vi "Populate Graph Channel Names.vi"(8 "error in (no error)":errorcluster, 10 "Array":string[](array[string]), 11 "WaveformGraph in":refnum<vi>) -> (0 "error out":errorcluster, 3 "WaveformGraph out":refnum<vi>)   [LabVIEW 2015, in "Utility.lvlib"]
uses:
  Utility.lvlib
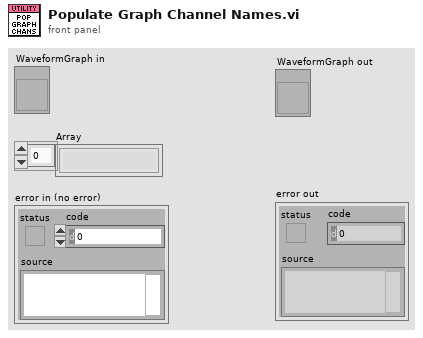
[diagram p1: front panel]
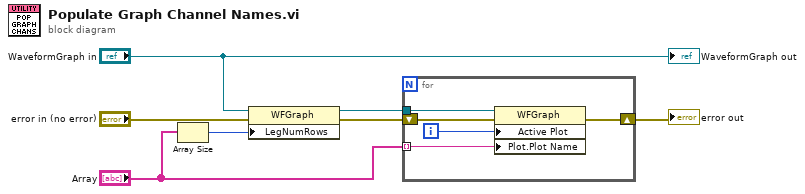
[diagram p0: block diagram]
diagram:
  n1 = Array Size(array="Array") -> (size(s)=w7:i32)
  n2 = property class="WFGraph"(reference="WaveformGraph in", error in="error in (no error)", "LegNumRows"=w7) -> (reference out=w5:refnum<vi>, error out=w3:errorcluster)
  n3 = for {
    tunnel: "Array" -> [w11] mode=indexing
    tunnel: w5 -> [w12]
    shift-right: [w8] -> w4
    shift-left: w3 -> [w9]
    i -> [w10]
    n4 = property class="WFGraph"(reference=w12, error in=w9, "Active Plot"=w10, "Plot.Plot Name"=w11) -> (error out=w8:errorcluster)  [unwired: 1 out]
  }
  "error out" <- w4
  "WaveformGraph out" <- "WaveformGraph in"
